vi "Test WSS Server.vi"() -> ()   [LabVIEW 2020]
uses:
  lv-http-util/HTTP Utils/Request/Request.lvclass
  lv-http-util/HTTP Utils/Response/Response.lvclass
  Stream-Websocket/Websocket Server/Websocket Server.lvclass
  lv-stream/stream/Endpoint/Endpoint.lvclass
  lv-stream/stream/Stream/Stream.lvclass
  Stream-Websocket/Websocket Client/Websocket Client.lvclass
panel:
  out "Last Client":refnum<k5>
  in  "HTTPS Port":u16=7080
  out "WSS":errorcluster
  out "HTTPS":errorcluster
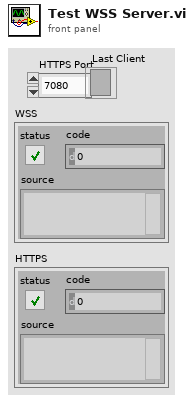
[diagram p1: front panel]
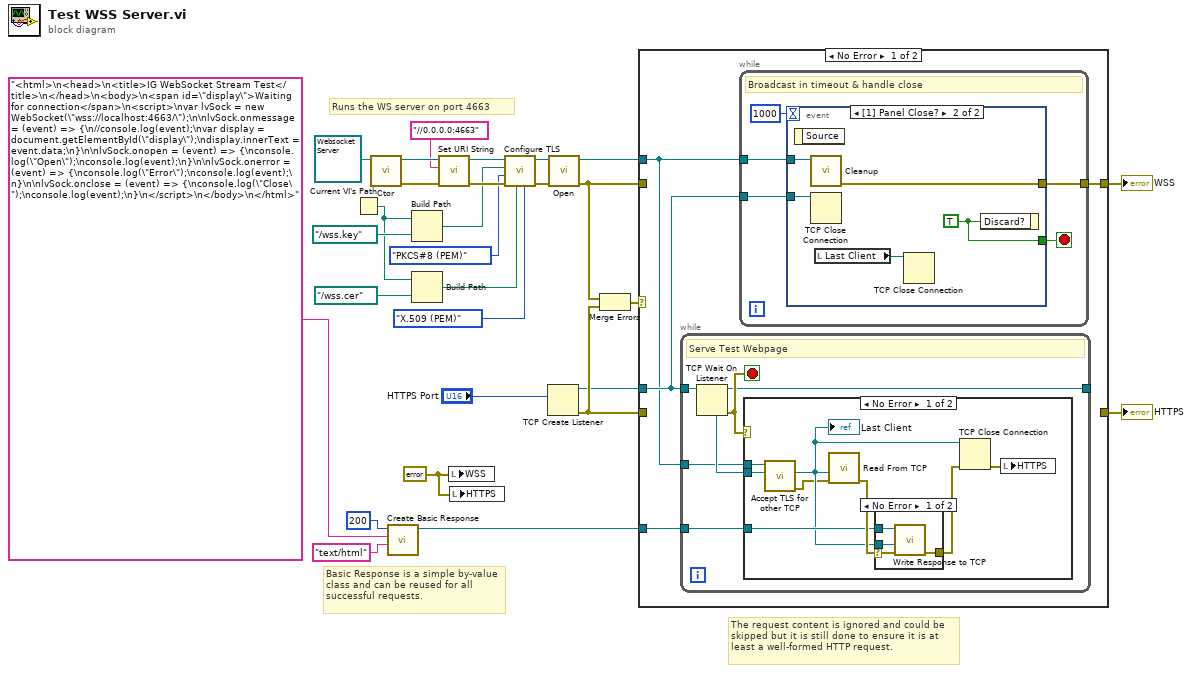
[diagram p0: block diagram]
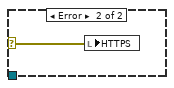
[diagram p3: hidden frame]
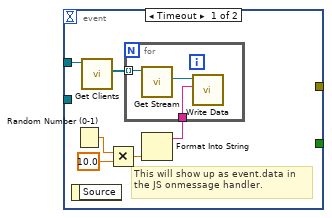
[diagram p4: hidden frame]
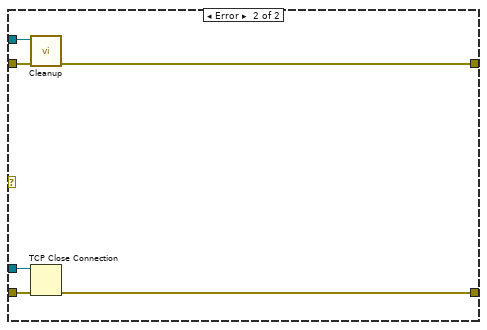
[diagram p5: hidden frame]
diagram:
  w18 = errorcluster {"status"=FALSE, "code"=0, "source"=""} ("WS")
  # "The request content is ignored and could be skipped but it is still done to ensure it is at least a well-formed HTTP request."
  # "Basic Response is a simple by-value class and can be reused for all successful requests."
  # "Runs the WS server on port 4663"
  n1 = Current VI's Path() -> (path=w4:path)
  n2 = call-dynamic "Ctor.vi"("Websocket Server in"=refnum<class "Websocket Server.lvclass"> refnum) -> ("error out"=w20:errorcluster, "Websocket Server out"=w22:refnum<class "Websocket Server.lvclass">)  [unwired: 9 in]
  n3 = call "Create Basic Response.vi"("Content-Type (text/plain)"="text/html", "Payload"="<html>\n<head>\n<title>IG WebSocket Stream Test</title>\n</head>\n<body>\n<span id=\"display\">Waiting for connection</span>\n<script>\nvar lvSock = new WebSocket(\"wss://localhost:4663/\");\n\nlvSock.onmessage = (event) => {\n//console.log(event);\nvar display = document.getElementById(\"display\");\ndisplay.innerText = event.data;\n}\n\nlvSock.onopen = (event) => {\nconsole.log(\"Open\");\nconsole.log(event);\n}\n\nlvSock.onerror = (event) => {\nconsole.log(\"Error\");\nconsole.log(event);\n}\n\nlvSock.onclose = (event) => {\nconsole.log(\"Close\");\nconsole.log(event);\n}\n</script>\n</body>\n</html>", "Status Code"=u16 200) -> ("Response out"=w25:refnum<class "Response.lvclass">)  [unwired: 7 in, 1 out]
  n4 = Build Path(base path=w4, name or relative path=path "../wss.key") -> (appended path=w6:path)
  n5 = Build Path(base path=w4, name or relative path=path "../wss.cer") -> (appended path=w3:path)
  n6 = call "Set URI String.vi"("error in (no error)"=w20, "URI String"="//0.0.0.0:4663", "Endpoint in"=w22) -> ("error out"=w10:errorcluster, "Endpoint out"=w11:refnum<class "Websocket Server.lvclass">)  [unwired: 7 in]
  n7 = local write "WSS"(w18) -> ()
  n8 = local write "HTTPS"(w18) -> ()
  n9 = call "Configure TLS.vi"("Cert Chain Format"=enum32{"X.509 (PEM)"}."X.509 (PEM)", "Cert Chain Path"=w3, "error in (no error)"=w10, "Private Key Format"=enum32{"PKCS#8 (PEM)", "PKCS#8 (DER)"}."PKCS#8 (PEM)", "Private Key Path"=w6, "Websocket Server in"=w11) -> ("error out"=w9:errorcluster, "Websocket Server out"=w8:refnum<class "Websocket Server.lvclass">)  [unwired: 4 in]
  n10 = TCP Create Listener(10:"HTTPS Port") -> (0:w28:errorcluster, 3:w16:refnum<k5>)  [unwired: 4 in, 1 out]
  n11 = call "Open.vi"("error in (no error)"=w9, "Endpoint in"=w8) -> ("error out"=w15:errorcluster, "Endpoint out"=w19:refnum<class "Websocket Server.lvclass">)  [unwired: 8 in]
  n12 = Merge Errors(w15, w28) -> (w14:errorcluster)
  n13 = case shown="No Error" w14 {
    tunnel: w25 -> [w32 _]
    tunnel: w19 -> [w29 w76]
    tunnel: w16 -> [w31 w74]
    tunnel: w15 -> [_ w77]
    tunnel: w28 -> [_ w73]
    tunnel: [_ w72] -> w13
    tunnel: [w30 w75] -> w12
    frame No Error {
      n14 = while {
        tunnel: w31 -> [w38]
        tunnel: w32 -> [w35]
        tunnel: [w34] -> _
        tunnel: w29 -> [w33]
        stop <- w37 stop-if-true
        # "Serve Test Webpage"
        n15 = TCP Wait On Listener(11:w38) -> (0:w37:errorcluster, 3:w34:refnum<k5>, 4:w36:refnum<k5>)  [unwired: 3 in, 2 out]
        n16 = case shown="No Error" w37 {
          selector: w37 -> [_ w52]
          tunnel: w36 -> [w42 _]
          tunnel: w35 -> [w44 _]
          tunnel: w33 -> [w39 _]
          frame No Error {
            n17 = call "Accept TLS for other TCP.vi"("TCP Connection In"=w42, "Websocket Server in"=w39) -> ("error out"=w40:errorcluster, "TCP Connection"=w41:refnum<k5>)  [unwired: 7 in, 1 out]
            "Last Client" <- w41
            n18 = call "Read From TCP.vi"("error in (no error)"=w40, "TCP Connection"=w41) -> ("error out"=w46:errorcluster)  [unwired: 8 in, 1 out]
            n19 = case shown="No Error" w46 {
              selector: w46 -> [w50 w51]
              tunnel: w44 -> [w49 _]
              tunnel: w41 -> [w48 _]
              tunnel: [w47 w51] -> w45
              frame No Error {
                n20 = call "Write Response to TCP.vi"("error in (no error)"=w50, "TCP Connection"=w48, "Response in"=w49) -> ("error out"=w47:errorcluster)  [unwired: 7 in, 1 out]
              }
              frame Error {
              }
            }
            n21 = TCP Close Connection(connection ID=w41, error in (no error)=w45) -> (error out=w43:errorcluster)  [unwired: 1 in, 1 out]
            n22 = local write "HTTPS"(w43) -> ()
          }
          frame Error {
            n23 = local write "HTTPS"(w52) -> ()
          }
        }
      }
      n24 = while {
        tunnel: w31 -> [w57]
        tunnel: w29 -> [w55]
        tunnel: [w53] -> w30
        stop <- w56 stop-if-true
        # "Broadcast in timeout & handle close"
        n25 = event shown="[1] Panel Close?" {
          selector: _ -> [_ _]
          dyn-events: _ -> [_ _]
          timeout: 1000 -> [_ _]
          tunnel: w57 -> [_ w71]
          tunnel: [_ w70] -> w56
          tunnel: w55 -> [w63 w69]
          tunnel: [_ w68] -> w53
          event Timeout {
            # "This will show up as event.data in the JS onmessage handler."
            n26 = event-data() -> ()  [unwired: 1 in, 1 out]
            n27 = Random Number (0-1)() -> (number: 0 to 1=w62:dbl)
            n28 = call "Get Clients.vi"("Websocket Server in"=w63) -> ("Clients"=w59:refnum<class "Websocket Client.lvclass">[])  [unwired: 8 in, 2 out]
            n29 = Multiply(x=w62, y=10.0) -> (x*y=w60:dbl)
            n30 = Format Into String(w60) -> (resulting string=w58:string)  [unwired: 3 in, 1 out]
            n31 = for {
              tunnel: w59 -> [w65] mode=indexing
              tunnel: w58 -> [w66]
              n32 = call-dynamic "Get Stream.vi"("Websocket Client in"=w65) -> ("Stream"=w64:refnum<class "Stream.lvclass">)  [unwired: 8 in, 2 out]
              n33 = call "Write Data.vi"("Data"=w66, "Stream in"=w64) -> ()  [unwired: 8 in, 2 out]
            }
          }
          event Panel Close? {
            w70 = TRUE ("Discard?")
            n34 = event-data() -> ()  [unwired: 1 in, 1 out]
            n35 = call-dynamic "Cleanup.vi"("Websocket Server in"=w69) -> ("error out"=w68:errorcluster)  [unwired: 10 in]
            n36 = TCP Close Connection(connection ID=w71) -> ()  [unwired: 2 in, 2 out]
            n37 = local read "Last Client"() -> (w67:refnum<k5>)
            n38 = TCP Close Connection(connection ID=w67) -> ()  [unwired: 2 in, 2 out]
            n39 = event-data("Discard?"=w70) -> ()  [unwired: 1 in, 1 out]
          }
        }
      }
    }
    frame Error {
      n40 = call-dynamic "Cleanup.vi"("error in (no error)"=w77, "Websocket Server in"=w76) -> ("error out"=w75:errorcluster)  [unwired: 9 in]
      n41 = TCP Close Connection(connection ID=w74, error in (no error)=w73) -> (error out=w72:errorcluster)  [unwired: 1 in, 1 out]
    }
  }
  "WSS" <- w12
  "HTTPS" <- w13
